vi "Analog Output.vi"(0 "VISA resource name":refnum<visa-resource-name>="GPIB0::16::INSTR", 5 "Output Channel(s) (123)":string="123", 9 "Output Voltage (0.0 V)":dbl, 11 "error in (no error)":errorcluster) -> (4 "VISA resource name out":refnum<visa-resource-name>, 15 "error out":errorcluster)   [LabVIEW 2020, in "Keithley 27XX.lvlib"]
doc: "This VI is used to set the analog output voltage on a selected line. \n\nNote\n(1) The Model 77xx card being used must support Analog Output to use this VI. \n\n(2) On the 7706 Multiplexer Card there are two 16-bit analog output channels - Ch 23 and Ch 24"
uses:
  Keithley 27XX.lvlib
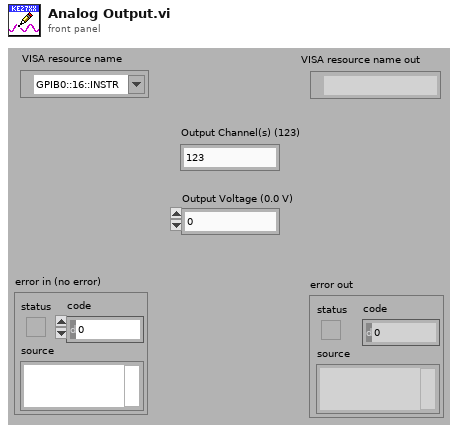
[diagram p1: front panel]
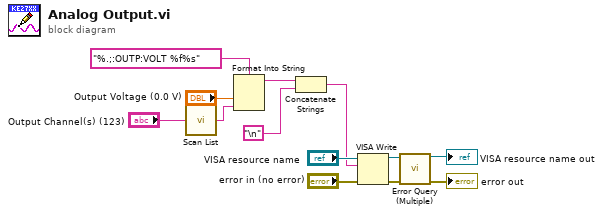
[diagram p0: block diagram]
diagram:
  n1 = call "Scan List.vi"("Scan List (Empty)"="Output Channel(s) (123)") -> ("Scan List Out"=w9:string)  [unwired: 14 in]
  n2 = Format Into String(format string="%.;:OUTP:VOLT %f%s", "Output Voltage (0.0 V)", w9) -> (resulting string=w3:string)  [unwired: 2 in, 1 out]
  n3 = Concatenate Strings(w3, "\n") -> (w1:string)
  n4 = VISA Write(VISA resource name="VISA resource name", write buffer=w1, error in (no error)="error in (no error)") -> (VISA resource name out=w7:refnum<visa-resource-name>, error out=w6:errorcluster)  [unwired: 1 out]
  n5 = call "Error Query (Multiple).vi"("VISA resource name"=w7, "error in (no error)"=w6) -> ("VISA resource name out"=→"VISA resource name out":refnum<visa-resource-name>, "error out"=→"error out":errorcluster)  [unwired: 10 in, 2 out]
